vi "MCCMSG Get Meter Irms Enable.vi"(8 "error in (no error)":errorcluster, 9 "pnError":i32, 10 "pbEnable":i32, 11 "hMCCmsg":i32) -> (0 "error out":errorcluster, 1 "pnError out":i32, 2 "pbEnable out":i32, 3 "function return":i32)   [LabVIEW 2012, in "MultiClamp 700B Controls.lvlib" / "AxMultiClampMsg.lvlib"]
doc: "AXMCCMSG BOOL WINAPI MCCMSG_GetMeterIrmsEnable(HMCCMSG hMCCmsg, BOOL *pbEnable, int *pnError);"
uses:
  AxMultiClampMsg.lvlib
  AxMultiClampMsg.dll
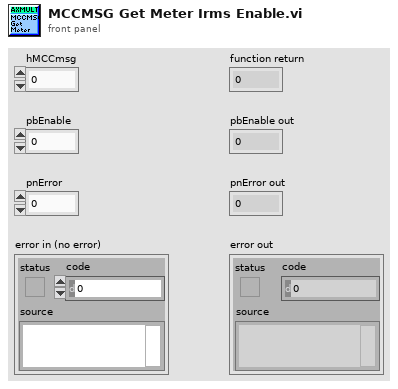
[diagram p1: front panel]
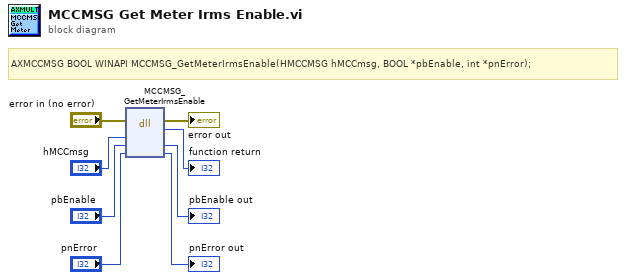
[diagram p0: block diagram]
diagram:
  # "AXMCCMSG BOOL WINAPI MCCMSG_GetMeterIrmsEnable(HMCCMSG hMCCmsg, BOOL *pbEnable, int *pnError);"
  n1 = dll-call lib="C:/Users/LAA12/Desktop/Rita/Multiclamp 700B VIs/AxMultiClampMsg/AxMultiClampMsg.*" fn="MCCMSG_GetMeterIrmsEnable"(error in="error in (no error)", "hMCCmsg"="hMCCmsg", "pbEnable"="pbEnable", "pnError"="pnError") -> (error out=→"error out":errorcluster, →"function return":i32, "pbEnable"=→"pbEnable out":i32, "pnError"=→"pnError out":i32)  [unwired: 3 in, 1 out]
